vi "ics_save_3D_2ch.vi"(0 "pixels":i32, 1 "filename":string, 3 "folder":path=path "D:/User/Sergey/ids_ics_trainer", 5 "Dwell":dbl, 7 "slices Z":i32, 9 "Range Z":dbl, 11 "Range":dbl, 12 "scale I":i32=1) -> (4 "saved":bool, 6 "path to .ids":path, 15 "error out":errorcluster)   [LabVIEW 2016]
panel:
  in  "error in":errorcluster
  out "text":string
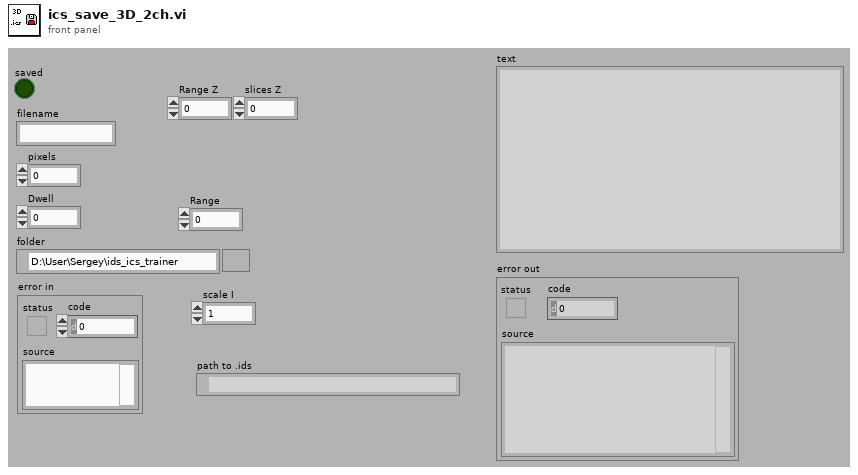
[diagram p1: front panel]
types:
  T1 = enum16{"open", "replace", "create", "open or create", "replace or create", "replace or create with confirmation"}
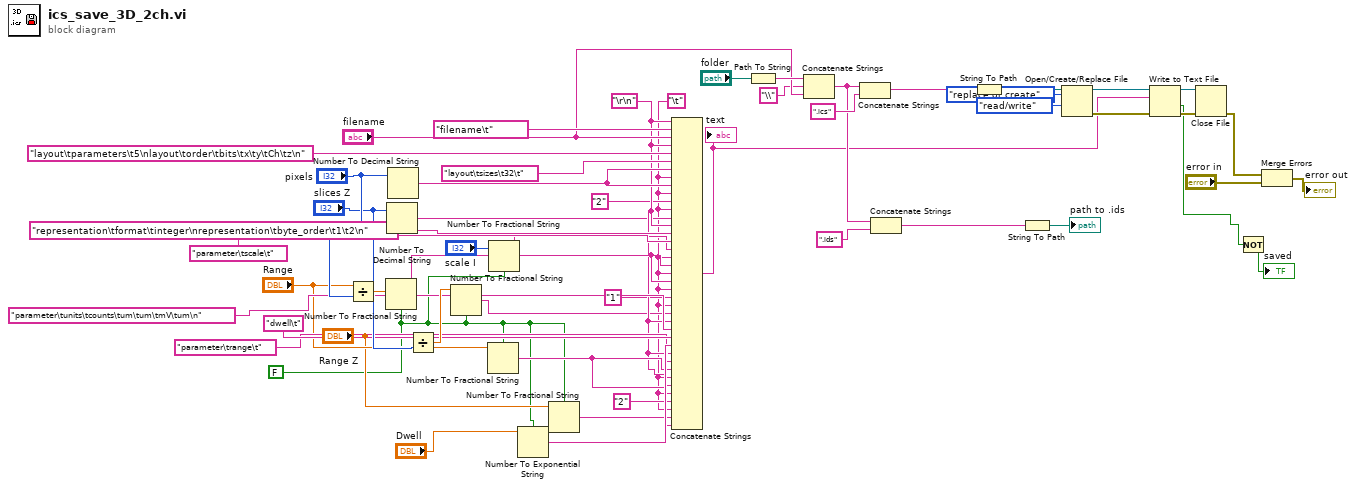
[diagram p0: block diagram]
diagram:
  w12 = FALSE ("use system decimal point (T)")
  w1 = "\t"
  w11 = "\r\n"
  n1 = Divide(x="Range", y="pixels") -> (x/y=w28:dbl)
  n2 = Number To Fractional String(use system decimal point (T)=w12, number=w28) -> (F-format string=w25:string)  [unwired: 2 in]
  n3 = Number To Decimal String(number="slices Z") -> (decimal integer string=w6:string)  [unwired: 1 in]
  n4 = Number To Decimal String(number="pixels") -> (decimal integer string=w32:string)  [unwired: 1 in]
  n5 = Divide(x="Range Z", y="slices Z") -> (x/y=w23:dbl)
  n6 = Number To Fractional String(use system decimal point (T)=w12, number=w23) -> (F-format string=w5:string)  [unwired: 2 in]
  n7 = Number To Fractional String(use system decimal point (T)=w12, number="Range") -> (F-format string=w16:string)  [unwired: 2 in]
  n8 = Number To Fractional String(use system decimal point (T)=w12, number="scale I") -> (F-format string=w26:string)  [unwired: 2 in]
  n9 = Number To Exponential String(number="Dwell", 1:w12) -> (E-format string=w19:string)  [unwired: 2 in]
  n10 = Number To Fractional String(use system decimal point (T)=w12, number="Range Z") -> (F-format string=w3:string)  [unwired: 2 in]
  n11 = Concatenate Strings(w11, "filename\t" ("string"), "filename", w11, "layout\tparameters\t5\nlayout\torder\tbits\tx\ty\tCh\tz\n" ("string"), "layout\tsizes\t32\t" ("string"), w32, w1, w32, w1, "2" ("string"), w1, w6, w11, "representation\tformat\tinteger\nrepresentation\tbyte_order\t1\t2\n" ("string"), "parameter\tscale\t" ("string"), w26, w1, w25, w1, w25, w1, "1" ("string"), w1, w5, w11, "parameter\tunits\tcounts\tum\tum\tmV\tum\n" ("string"), "dwell\t" ("string"), w19, w11, "parameter\trange\t" ("string"), w16, w1, w16, w1, "2" ("string"), w1, w3, w11) -> (w37:string)
  "text" <- w37
  n12 = Path To String(path="folder") -> (string=w46:string)
  n13 = Concatenate Strings(w46, "\\" ("string"), "filename") -> (w39:string)
  n14 = Concatenate Strings(w39, ".ics" ("string")) -> (w41:string)
  n15 = Concatenate Strings(w39, ".ids" ("string")) -> (w38:string)
  n16 = String To Path(string=w41) -> (path=w45:path)
  n17 = String To Path(string=w38) -> (path=→"path to .ids":path)
  n18 = Open/Create/Replace File(file path (use dialog)=w45, operation (0:open)=T1."replace or create", access (0:read/write)=enum16{"read/write", "read-only", "write-only"}."read/write") -> (refnum out=w48:refnum<file>, error out=w47:errorcluster)  [unwired: 3 in, 1 out]
  n19 = Write to Text File(file (use dialog)=w48, text=w37, error in=w47) -> (refnum out=w50:refnum<file>, cancelled=w10:bool, error out=w49:errorcluster)  [unwired: 1 in]
  n20 = Close File(refnum=w50, error in=w49) -> (error out=w36:errorcluster)  [unwired: 1 out]
  n21 = Not(x=w10) -> (.not. x?=→"saved":bool)
  n22 = Merge Errors(w36, "error in") -> (→"error out":errorcluster)
